vi "satellite simulator control.vi"() -> ()   [LabVIEW 2012]
uses:
  <vilib>/Utility/error.llb/DialogType.ctl
  <vilib>/DAQmx/create/channels.llb/DAQmx Create Channel (DO-Digital Output).vi
  <vilib>/Instr/_visa.llb/VISA Configure Serial Port (Instr).vi
  <vilib>/vision/NI_Vision_Development_Module.lvlib
  <vilib>/ptbypt/NI_PtbyPt.lvlib
panel:
  in  "Reaction Wheel":bool
  out "Write String":string
  in  "Control Value":sgl=1.5 format="%.4f"
  in  "Control Mode":u16(ring) items=["Idle"=0, "PWM (-1..1)"=1, "Current (-2.5..2.5A)"=2, "Speed (Rads/s)"=3, "Acceleration (Rads/sec^2)"=16, "Momentum (N-m-sec)"=17, "Torque (N-m)"=18]
  in  "Dst":i32=36 format="%x"
  in  "stop bits":u16(ring)=10 items=["1.0"=10, "1.5"=15, "2.0"=20]
  in  "VISA resource name (write)":refnum<visa-resource-name>="COM4"
  in  "flow control":u16(ring) items=["None"=0, "XON/XOFF"=1, "RTS/CTS"=2, "DTR/DSR"=4]
  in  "parity (0:none)":u16(ring) items=["None", "Odd", "Even", "Mark", "Space"]
  in  "data bits (8)":u16=8 min=5 max=8 step=1
  in  "baud rate (115200)":u32=115200
  out "bytes written":u32
  in  "bytes to read":u32=12
  out "Read string":string
  out "bytes read":u32
  out "Filtered Ohmega":dbl format="%0.2f"
  in  "VISA resource name":refnum<visa-resource-name>
  out "read buffer":string
  out "Ohmega":dbl[](graph)
  out "Filtered Ohmega":dbl[](graph)
  in  "Floating":bool
  in  "Thruster 8":bool
  in  "Thruster 7":bool
  in  "Thruster 6":bool
  in  "Thruster 5":bool
  in  "Thruster 4":bool
  in  "Thruster 3":bool
  in  "Thruster 2":bool
  in  "Truster1":bool
  in  "Thrusters Bundled":bool=TRUE
  in  "Manual Control Mode (Default)":bool
  in  "Up":bool
  in  "Right":bool
  in  "Down":bool
  in  "Left":bool
  in  "Stop 2":bool
  in  "CntrClk":bool
  in  "ClkWise":bool
  in  "Angular Acceleration":u16(ring) items=["Fast", "Slow"]
  in  "Duty Cycle":dbl=1.0
  in  "Automatic PD Position Controller":bool
  in  "Pixel-Distance Ratio (pix/cm)":dbl=8.26
  in  "Remote Logger Status":bool
  in  "Downlink Object Data?":bool
  in  "Remote Port":u16=61557
  in  "Local Port":u16=61556
  in  "Remote Host":string="localhost"
  in  "broadcast":bool
  in  "Maintain Attitude":bool
  out "alpha":dbl
  out "Objects":T1(array[cluster]) {"Aspect Ratio" format="%.2f"; "Orientation" format="%.2f"; "Area" format="%.2f"; "Object Center"."Y" format="%.2f"; "Object Center"."X" format="%.2f"}
  in  "Y Center Correction":dbl
  in  "X Center Correction":dbl
  out "Offset Degree":dbl
  in  "Y Desired":dbl
  in  "X Desired":dbl
  out "Vx (cm/s)":dbl
  out "Vy (cm/s)":dbl
  in  "OK Button":bool
  in  "Air Floating Status":bool
  in  "Control Freq":u32=20
  in  "Alpha Desired":dbl
  in  "STOP":bool caption="stop (F)"
  out "Image Out":T2(plugin-control)
  out "alpha (deg)":dbl
  out "dx (cm)":dbl
  out "dy (cm)":dbl
  # "Bundled Operations"
  # "Unbundled Operations"
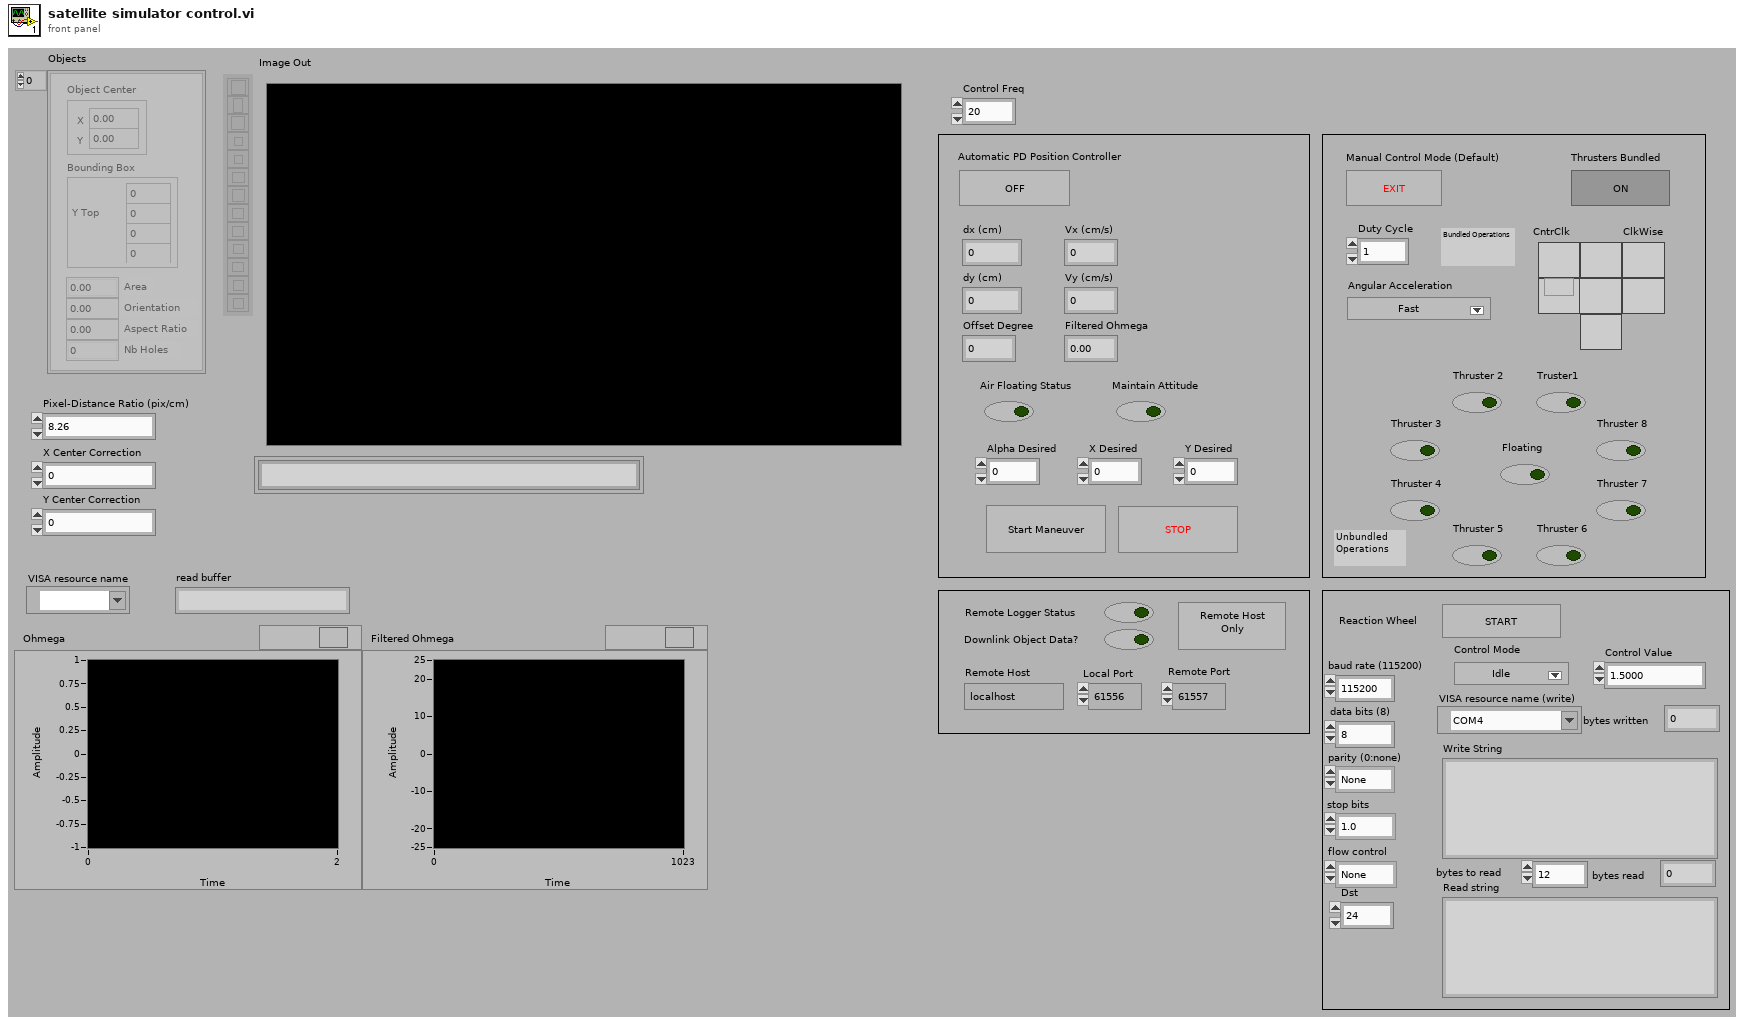
[diagram p1: front panel]
types:
  T1 = cluster{"Object Center":cluster{"X":sgl, "Y":sgl}, "Bounding Box":cluster{"X Left":i32, "Y Top":i32, "X Right":i32, "Y Bottom":i32}, "Area":sgl, "Orientation":sgl, "Aspect Ratio":sgl, "Nb Holes":i32}[]
  T2 = typedef "IMAQ Image.ctl" = refnum<image>
  T3 = typedef "DialogType.ctl" = u16
  T4 = cluster{"dx (cm)":dbl, "dy (cm)":dbl, "Offset Degree":dbl}
  T5 = cluster{"Objects":u16, "Threshold":i32, "Reject Border":bool, "Fill Holes":bool, "Min Object Size":bool, "Min Size":i32, "Max Object Size":bool, "Max Size":i32, "Show Search Area":bool, "Show Center":bool, "Show Bounding Box":bool}
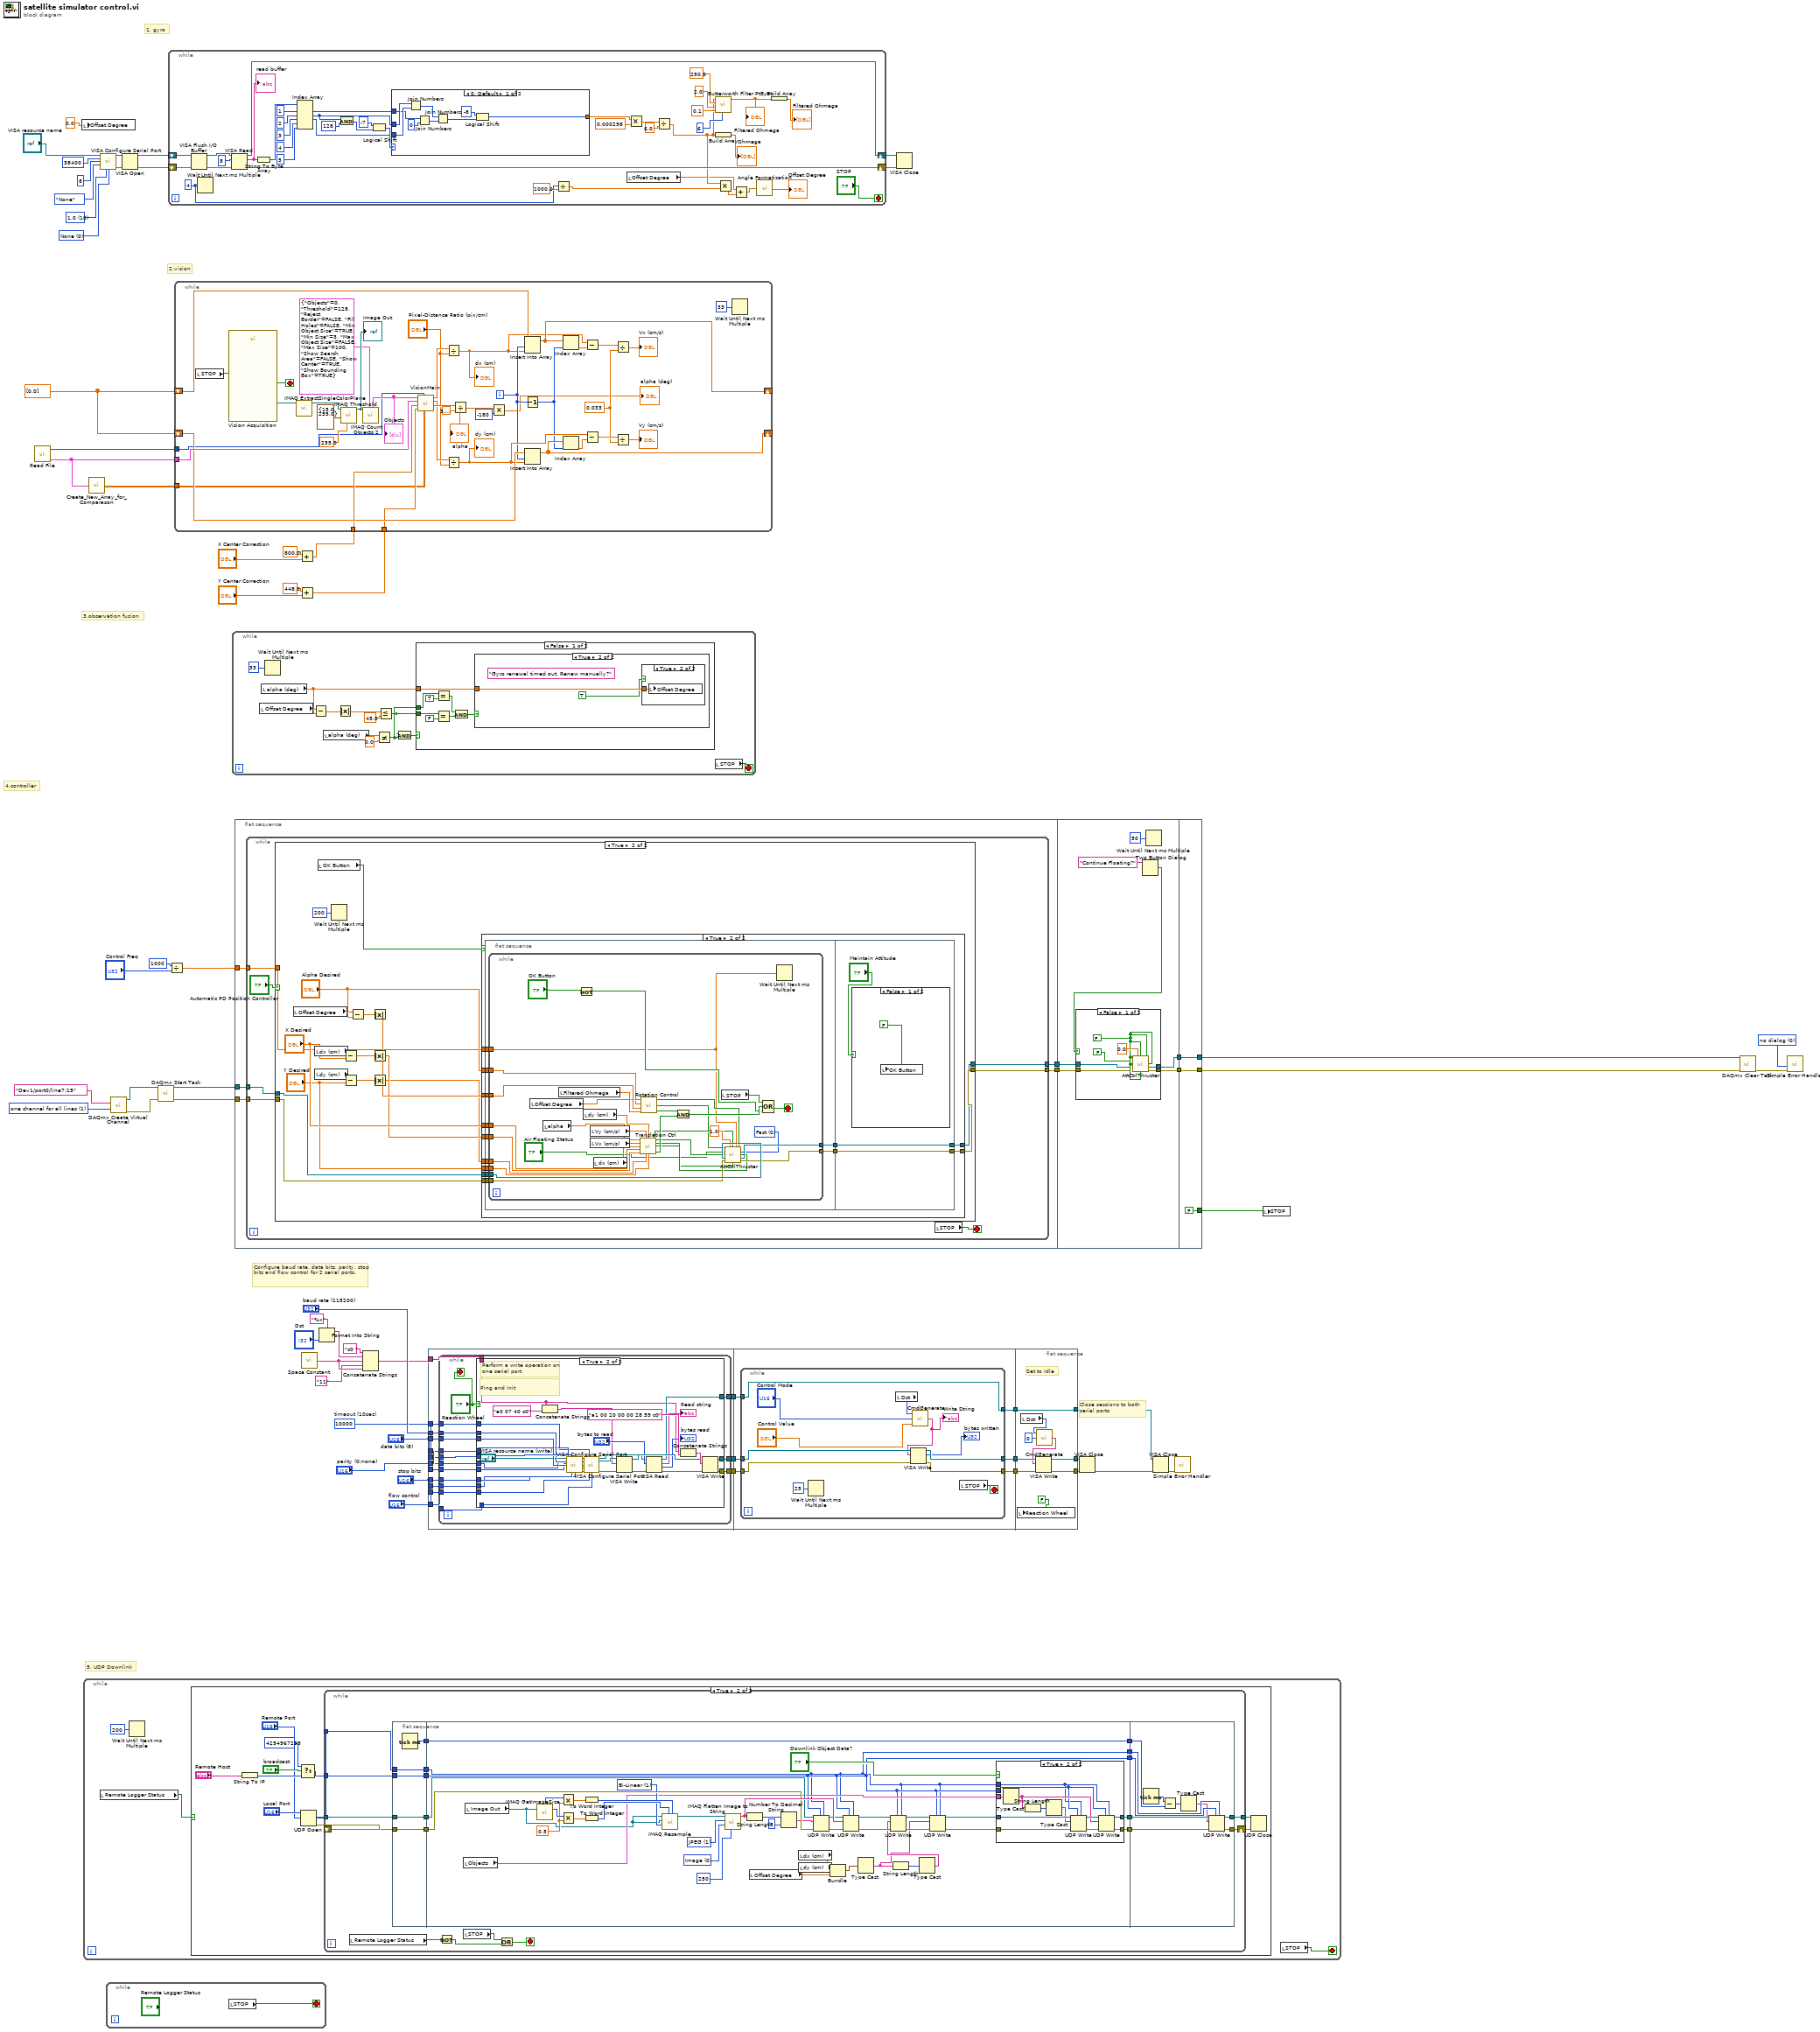
[diagram p0: block diagram]
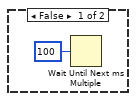
[diagram p2: hidden frame]
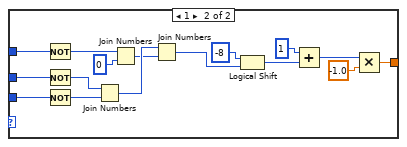
[diagram p3: hidden frame]
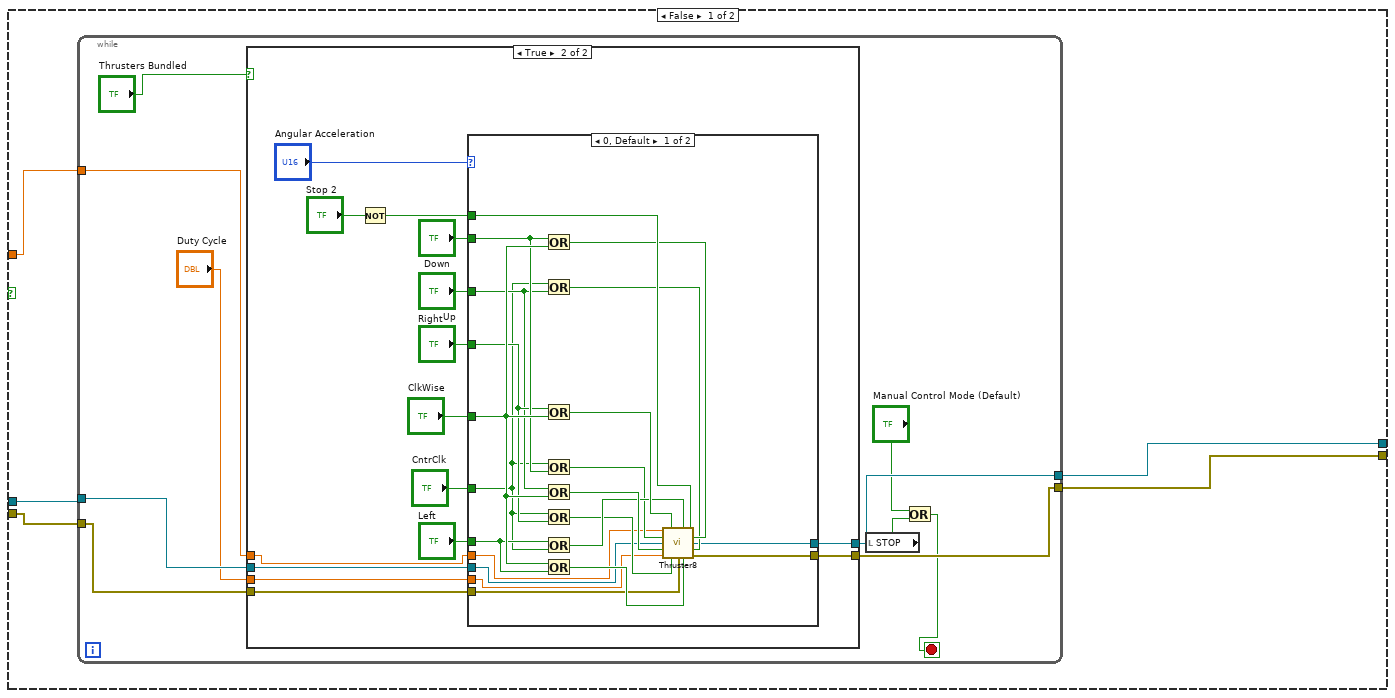
[diagram p6: hidden frame]
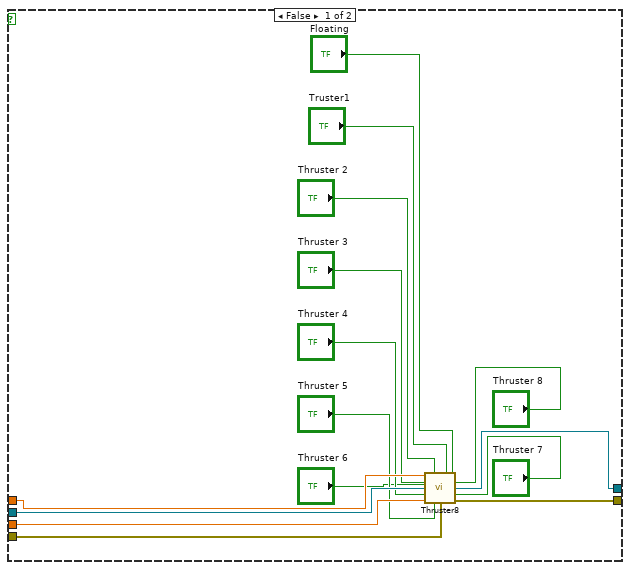
[diagram p7: hidden frame]
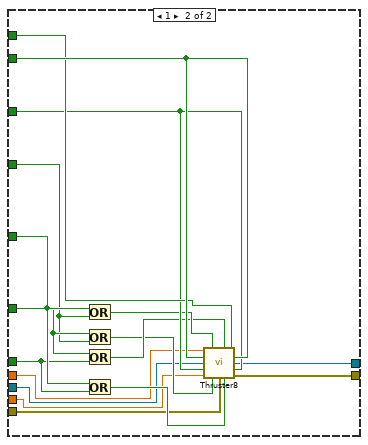
[diagram p8: hidden frame]
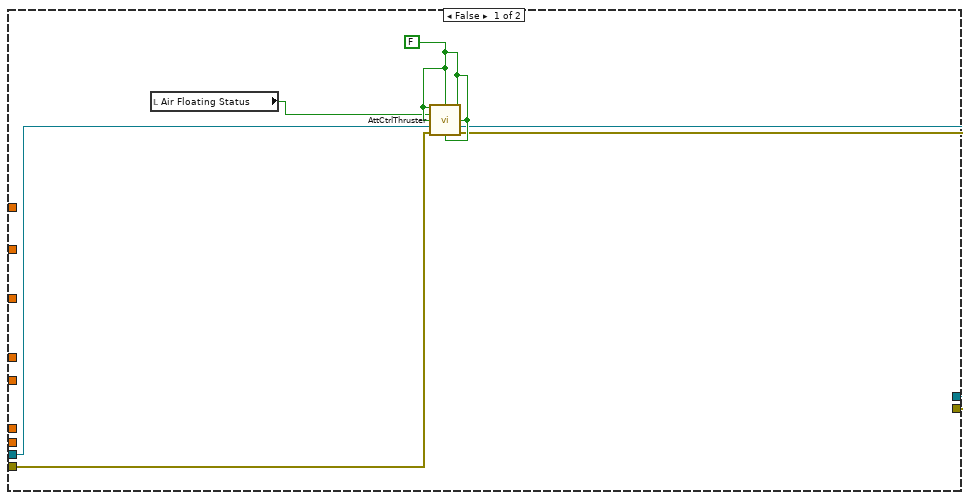
[diagram p9: hidden frame]
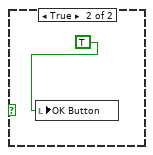
[diagram p10: hidden frame]
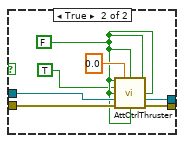
[diagram p11: hidden frame]
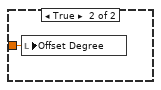
[diagram p14: hidden frame]
diagram:
  w15 = u32 10000  # timeout (10sec)
  w30 = u16 0 items=["None", "XON/XOFF", "RTS/CTS", "XON/XOFF & RTS/CTS", "DTR/DSR", "XON/XOFF & DTR/DSR"] ("flow control (0:none)")
  w32 = u16 10 items=["1.0"=10, "1.5"=15, "2.0"=20] ("stop bits (10: 1 bit)")
  w60 = T3 0 items=["no dialog", "OK message", "continue or stop message", "OK message + warnings", "continue/stop + warnings"] ("type of dialog (OK msg:1)")
  w63 = 1 items=["one channel for each line", "one channel for all lines"] ("line grouping")
  w49 = dbl[] [0.0]
  # "Close sessions to both serial ports"
  # "Configure baud rate, data bits, parity, stop bits and flow control for 2 serial ports."
  # "5. UDP Downlink"
  # "4.controller"
  # "3.observation fusion"
  # "2.vision"
  # "1. gyro"
  n1 = call "Read File.vi"() -> ("Objects"=w29:T1, "Total Obj"=w27:i32)  [unwired: 1 in]
  n2 = local write "Offset Degree"(0.0 ("y")) -> ()
  n3 = while {
    stop <- w67 stop-if-true
    n4 = local read "Remote Logger Status"() -> (w68:bool)
    n5 = Wait Until Next ms Multiple(millisecond multiple=u32 200) -> ()  [unwired: 1 out]
    n6 = case shown="True" w68 {
      frame False {
      }
      frame True {
        n7 = String To IP(1:"Remote Host") -> (0:w76:u32)
        n8 = Select(t=u32 4294967295, s="broadcast", f=w76) -> (s? t:f=w73:u32)
        n9 = UDP Open(11:"Local Port") -> (port=w72:refnum<k16>, 0:w71:errorcluster)  [unwired: 1 in, 4 out]
        n10 = while {
          tunnel: "Remote Port" -> [w99]
          tunnel: w73 -> [w98]
          tunnel: w72 -> [w97]
          tunnel: [w95] -> w70
          shift-right: [w94] -> w69
          shift-left: w71 -> [w96]
          stop <- w83 stop-if-true
          n11 = local read "Remote Logger Status"() -> (w81:bool)
          n12 = flat-sequence {
            tunnel: w97 -> [w101]
            tunnel: w99 -> [w102]
            tunnel: w98 -> [w103]
            tunnel: w96 -> [w104]
            tunnel: [w104] -> w93
            tunnel: [w103] -> w92
            tunnel: [w102] -> w91
            tunnel: [w101] -> w90
            tunnel: [w100] -> w89
            tunnel: [w124] -> w88
            tunnel: [w123] -> w87
            tunnel: w93 -> [w142]
            tunnel: w92 -> [w106]
            tunnel: w91 -> [w105]
            tunnel: w90 -> [w126]
            tunnel: [w125] -> w86
            tunnel: w89 -> [w125]
            tunnel: [w105] -> w85
            tunnel: [w106] -> w84
            tunnel: [w166] -> w95
            tunnel: [w160] -> w94
            tunnel: w88 -> [w161]
            tunnel: w87 -> [w167]
            tunnel: w86 -> [w168]
            tunnel: w85 -> [w165]
            tunnel: w84 -> [w164]
            frame #0 {
              n13 = Tick Count (ms)() -> (millisecond timer value=w100:u32)
            }
            frame #1 {
              w130 = u32 1 items=["Zero Order", "Bi-Linear", "Quadratic", "Cubic Spline"] ("Interpolation Type")
              w131 = 0.5
              w139 = 0 items=["Image", "Image and Vision Info", "Reference to Image"] ("Type of Flatten (Image and Vision Info)")
              w144 = 1 items=["None", "JPEG", "PACKED BINARY"] ("Compression (None)")
              n14 = local read "Objects"() -> (w121:T1)
              n15 = local read "Image Out"() -> (w120:T2)
              n16 = call "IMAQ GetImageSize"("Image"=w120) -> ("Y Resolution"=w132:i32, "X Resolution"=w133:i32)  [unwired: 3 in, 1 out]
              n17 = Multiply(x=w133, y=w131) -> (x*y=w135:dbl)
              n18 = Multiply(x=w132, y=w131) -> (x*y=w137:dbl)
              n19 = To Word Integer(number=w135) -> (16bit integer=w134:i16)
              n20 = To Word Integer(number=w137) -> (16bit integer=w136:i16)
              n21 = call "IMAQ Resample"("X Resolution"=w134, "Y Resolution"=w136, "Interpolation Type"=w130, "Image Dst"=w120, "Image Src"=w120) -> ("Image Dst Out"=w138:T2)  [unwired: 5 in, 1 out]
              n22 = call "IMAQ Flatten Image to String"("Quality (750)"=250, "Type of Flatten (Image and Vision Info)"=w139, "Compression (None)"=w144, "Image"=w138) -> ("Data String"=w143:string)  [unwired: 6 in, 1 out]
              n23 = String Length(string=w143) -> (length=w129:i32)
              n24 = local read "Offset Degree"() -> (w117:dbl)
              n25 = Number To Decimal String(number=w129, width (-)=i16 5) -> (decimal integer string=w128:string)
              n26 = local read "dx (cm)"() -> (w119:dbl)
              n27 = local read "dy (cm)"() -> (w118:dbl)
              n28 = UDP Write(address=w106, port or service name=w105, connection ID=w126, data in=w128, 8:w142) -> (error out=w141:errorcluster, 3:w140:refnum<k16>)  [unwired: 1 out]
              n29 = Bundle("dx (cm)"=w119, "dy (cm)"=w118, "Offset Degree"=w117) -> (w116:T4)  [unwired: 1 in]
              n30 = UDP Write(address=w106, port or service name=w105, connection ID=w140, data in=w143, 8:w141) -> (error out=w114:errorcluster, 3:w115:refnum<k16>)  [unwired: 1 out]
              n31 = Type Cast(x=w116) -> (*(type *) &x=w107:string)  [unwired: 1 in]
              n32 = String Length(string=w107) -> (length=w109:i32)
              n33 = Type Cast(x=w109) -> (*(type *) &x=w108:string)  [unwired: 1 in]
              n34 = UDP Write(address=w106, port or service name=w105, connection ID=w115, data in=w108, 8:w114) -> (error out=w113:errorcluster, 3:w111:refnum<k16>)  [unwired: 1 out]
              n35 = UDP Write(address=w106, port or service name=w105, connection ID=w111, data in=w107, 8:w113) -> (error out=w112:errorcluster, 3:w110:refnum<k16>)  [unwired: 1 out]
              n36 = case shown="True" "Downlink Object Data?" {
                tunnel: w121 -> [_ w159]
                tunnel: w112 -> [w147 w157]
                tunnel: [w147 w155] -> w124
                tunnel: w110 -> [w146 w154]
                tunnel: [w146 w152] -> w123
                tunnel: w106 -> [_ w149]
                tunnel: w105 -> [_ w148]
                frame False {
                }
                frame True {
                  n37 = Type Cast(x=w159) -> (*(type *) &x=w150:string)  [unwired: 1 in]
                  n38 = String Length(string=w150) -> (length=w158:i32)
                  n39 = Type Cast(x=w158) -> (*(type *) &x=w151:string)  [unwired: 1 in]
                  n40 = UDP Write(address=w149, port or service name=w148, connection ID=w154, data in=w151, 8:w157) -> (error out=w156:errorcluster, 3:w153:refnum<k16>)  [unwired: 1 out]
                  n41 = UDP Write(address=w149, port or service name=w148, connection ID=w153, data in=w150, 8:w156) -> (error out=w155:errorcluster, 3:w152:refnum<k16>)  [unwired: 1 out]
                }
              }
            }
            frame #2 {
              n42 = Tick Count (ms)() -> (millisecond timer value=w169:u32)
              n43 = Subtract(x=w169, y=w168) -> (x-y=w163:u32)
              n44 = Type Cast(x=w163) -> (*(type *) &x=w162:string)  [unwired: 1 in]
              n45 = UDP Write(address=w164, port or service name=w165, connection ID=w167, data in=w162, 8:w161) -> (error out=w160:errorcluster, 3:w166:refnum<k16>)  [unwired: 1 out]
            }
          }
          n46 = Not(x=w81) -> (.not. x?=w80:bool)
          n47 = local read "STOP"() -> (w82:bool)
          n48 = Or(x=w82, y=w80) -> (x .or. y?=w83:bool)
        }
        n49 = UDP Close(connection ID=w70, 8:w69) -> ()  [unwired: 2 out]
      }
    }
    n50 = local read "STOP"() -> (w67:bool)
  }
  n51 = call "Create_New_Array_for_Comparason.vi"("Captured Plots"=w29) -> ("Generated Distance Array"=w28:dbl[][])
  n52 = call-poly "VISA Configure Serial Port"("VISA resource name"="VISA resource name", "baud rate (9600)"=u32 38400, "data bits (8)"=u16 8, "parity (0:none)"=enum16{"None", "Odd", "Even", "Mark", "Space"}."None", "stop bits (10: 1 bit)"=w32, "flow control (0:none)"=w30) -> ("VISA resource name out"=w37:refnum<visa-resource-name>, "error out"=w36:errorcluster)  [unwired: 8 in]
  n53 = while {
    stop <- w170 stop-if-true
    n54 = local read "STOP"() -> (w170:bool)
  }
  n55 = call-poly <vilib>:"DAQmx Create Virtual Channel.vi"("lines"=tag "Dev1/port0/line7:15" ("Lines"), "line grouping"=w63) -> ("task out"=w61:refnum<k21>, "error out"=w62:errorcluster)  [unwired: 12 in]
  n56 = VISA Open(error in (no error)=w36, VISA resource name=w37) -> (VISA resource name=w35:refnum<visa-resource-name>, error out=w34:errorcluster)  [unwired: 3 in]
  n57 = call <vilib>:"DAQmx Start Task.vi"("task/channels in"=w61, "error in"=w62) -> ("task out"=w56:refnum<k21>, "error out"=w55:errorcluster)  [unwired: 12 in]
  n58 = while {
    shift-right: [w180] -> w3
    shift-left: w34 -> [w209]
    shift-right: [w181] -> w4
    shift-left: w35 -> [w210]
    stop <- "STOP" stop-if-true
    w172 = u32 4 ("millisecond multiple")
    n59 = VISA Flush I/O Buffer(VISA resource name=w210, error in (no error)=w209) -> (VISA resource name out=w208:refnum<visa-resource-name>, error out=w207:errorcluster)  [unwired: 1 in]
    n60 = Wait Until Next ms Multiple(millisecond multiple=w172) -> ()  [unwired: 1 out]
    n61 = VISA Read(VISA resource name=w208, byte count=u32 8, error in (no error)=w207) -> (VISA resource name out=w181:refnum<visa-resource-name>, read buffer=w182:string, error out=w180:errorcluster)  [unwired: 1 out]
    "read buffer" <- w182
    n62 = String To Byte Array(string=w182) -> (unsigned byte array=w203:u8[])
    n63 = Index Array(array=w203, index #1=1 ("index"), index #2=2 ("index"), index #3=3 ("index"), index #4=4 ("index"), index #5=5 ("index")) -> (element #1=w187:u8, element #2=w186:u8, element #3=w185:u8)  [unwired: 2 out]
    n64 = And(x=w186, y=u8 128) -> (x .and. y?=w197:u8)
    n65 = Logical Shift(y=i16 -7, x=w197) -> (x << y=w195:u8)
    n66 = case shown="0, Default" w195 {
      tunnel: [w212 w221] -> w199
      tunnel: w187 -> [w213 w231]
      tunnel: w186 -> [w215 w230]
      tunnel: w185 -> [w214 w229]
      frame 0, Default {
        n67 = Join Numbers(hi=w215, lo=w214) -> ((hi.lo)=w220:u16)
        n68 = Join Numbers(hi=w213, lo=u8 0) -> ((hi.lo)=w218:u16)
        n69 = Join Numbers(hi=w220, lo=w218) -> ((hi.lo)=w217:u32)
        n70 = Logical Shift(y=i16 -8, x=w217) -> (x << y=w212:u32)
      }
      frame 1 {
        n71 = Not(x=w231) -> (.not. x?=w226:u8)
        n72 = Not(x=w230) -> (.not. x?=w228:u8)
        n73 = Not(x=w229) -> (.not. x?=w227:u8)
        n74 = Join Numbers(hi=w228, lo=w227) -> ((hi.lo)=w236:u16)
        n75 = Join Numbers(hi=w226, lo=u8 0) -> ((hi.lo)=w234:u16)
        n76 = Join Numbers(hi=w236, lo=w234) -> ((hi.lo)=w233:u32)
        n77 = Logical Shift(y=i16 -8, x=w233) -> (x << y=w225:u32)
        n78 = Add(x=u32 1, y=w225) -> (x+y=w222:u32)
        n79 = Multiply(x=w222, y=-1.0) -> (x*y=w221:dbl)
      }
    }
    n80 = Divide(x=w172, y=1000.0) -> (x/y=w171:dbl)
    n81 = local read "Offset Degree"() -> (w177:dbl)
    n82 = Multiply(x=w199, y=0.000298) -> (x*y=w205:dbl)
    n83 = Divide(x=w205, y=6.0) -> (x/y=w178:dbl)
    n84 = call <vilib>:"Butterworth Filter PtByPt.vi"("order"=6, "low cutoff freq: fl"=0.1, "high cutoff freq: fh"=2.0, "sampling freq: fs"=250.0, "x"=w178) -> ("Filtered x"=w189:dbl)  [unwired: 4 in, 1 out]
    "Filtered Ohmega" <- w189
    n85 = Build Array(w178) -> (→"Ohmega":dbl[])
    n86 = Multiply(x=w178, y=w171) -> (x*y=w176:dbl)
    n87 = Add(x=w177, y=w176) -> (x+y=w175:dbl)
    n88 = call "Angle Formatization.vi"("Alpha"=w175) -> ("Alpha Formatized"=→"Offset Degree":dbl)
    n89 = Build Array(w189) -> (→"Filtered Ohmega":dbl[])
  }
  n90 = Divide(x=u32 1000 ("milliseconds to wait"), y="Control Freq") -> (x/y=w52:dbl)
  n91 = while {
    stop <- w247 stop-if-true
    n92 = local read "Offset Degree"() -> (w246:dbl)
    n93 = local read "alpha (deg)"() -> (w242:dbl)
    n94 = Wait Until Next ms Multiple(millisecond multiple=u32 33) -> ()  [unwired: 1 out]
    n95 = Subtract(x=w246, y=w242) -> (x-y=w245:dbl)
    n96 = local read "alpha (deg)"() -> (w240:dbl)
    n97 = Absolute Value(x=w245) -> (abs(x)=w244:dbl)
    n98 = Not Equal?(x=w240, y=0.0) -> (x != y?=w238:bool)
    n99 = Less Or Equal?(x=w244, y=45.0) -> (x <= y?=w237:bool)
    n100 = And(x=w237, y=w238) -> (x .and. y?=w241:bool)
    n101 = case shown="False" w241 {
      tunnel: w242 -> [w249 w260]
      tunnel: w238 -> [w251 _]
      tunnel: w237 -> [w250 _]
      frame False {
        n102 = Equal?(x=w251, y=TRUE) -> (x = y?=w255:bool)
        n103 = Equal?(x=w250, y=FALSE) -> (x = y?=w254:bool)
        n104 = And(x=w255, y=w254) -> (x .and. y?=w252:bool)
        n105 = case shown="True" w252 {
          tunnel: w249 -> [_ w258]
          frame False {
          }
          frame True {
            (unwired) "Gyro renewal timed out. Renew manually?" ("message")
            n106 = case shown="True" TRUE {
              tunnel: w258 -> [_ w259]
              frame False {
              }
              frame True {
                n107 = local write "Offset Degree"(w259) -> ()
              }
            }
          }
        }
      }
      frame True {
        n108 = local write "Offset Degree"(w260) -> ()
      }
    }
    n109 = local read "STOP"() -> (w247:bool)
  }
  n110 = flat-sequence {
    tunnel: w56 -> [w265]
    tunnel: w55 -> [w264]
    tunnel: w52 -> [w261]
    tunnel: [w263] -> w51
    tunnel: [w262] -> w50
    tunnel: w51 -> [w450]
    tunnel: w50 -> [w448]
    tunnel: [w449] -> w42
    tunnel: [w447] -> w41
    tunnel: [w466] -> w53
    tunnel: [w467] -> w54
    tunnel: w42 -> [w467]
    tunnel: w41 -> [w466]
    tunnel: [FALSE] -> w40
    frame #0 {
      n111 = while {
        tunnel: w265 -> [w272]
        tunnel: w264 -> [w271]
        tunnel: [w270] -> w263
        tunnel: [w269] -> w262
        tunnel: w261 -> [w267]
        stop <- w268 stop-if-true
        n112 = case shown="True" "Automatic PD Position Controller" {
          tunnel: w272 -> [w276 w374]
          tunnel: w271 -> [w275 w373]
          tunnel: [w273 w372] -> w270
          tunnel: [w274 w371] -> w269
          tunnel: w267 -> [w277 w357]
          frame False {
            n113 = while {
              tunnel: w277 -> [w287]
              tunnel: w276 -> [w286]
              tunnel: [w285] -> w274
              tunnel: [w284] -> w273
              tunnel: w275 -> [w283]
              stop <- w280 stop-if-true
              n114 = case shown="True" "Thrusters Bundled" {
                tunnel: w287 -> [w298 w310]
                tunnel: w286 -> [w302 w309]
                tunnel: [w299 w308] -> w285
                tunnel: [w300 w307] -> w284
                tunnel: w283 -> [w301 w306]
                tunnel: "Duty Cycle" -> [w297 w303]
                frame False {
                  n115 = call "Thruster8.vi"("period"=w298, "Thruster 2"="Thruster 2", "Truster1"="Truster1", "Floating"="Floating", "Thruster 3"="Thruster 3", "Thruster 8"="Thruster 8", "task in"=w302, "Thruster 4"="Thruster 4", "Thruster 7"="Thruster 7", "Duty Cycle"=w297, "Thruster 5"="Thruster 5", "error in"=w301, "Thruster 6"="Thruster 6") -> ("task out"=w299:refnum<k21>, "error out"=w300:errorcluster)  [unwired: 1 in]
                }
                frame True {
                  n116 = Not(x="Stop 2") -> (.not. x?=w304:bool)
                  n117 = case shown="0, Default" "Angular Acceleration" {
                    tunnel: w304 -> [w338 w354]
                    tunnel: "Down" -> [w330 w355]
                    tunnel: "Left" -> [w332 w348]
                    tunnel: "Up" -> [w326 w353]
                    tunnel: "Right" -> [w328 w346]
                    tunnel: "ClkWise" -> [w334 w352]
                    tunnel: "CntrClk" -> [w325 w349]
                    tunnel: w303 -> [w323 w344]
                    tunnel: w310 -> [w322 w343]
                    tunnel: w309 -> [w321 w339]
                    tunnel: [w320 w340] -> w308
                    tunnel: [w319 w341] -> w307
                    tunnel: w306 -> [w318 w342]
                    frame 0, Default {
                      n118 = Or(x=w330, y=w334) -> (x .or. y?=w333:bool)
                      n119 = Or(x=w325, y=w326) -> (x .or. y?=w324:bool)
                      n120 = Or(x=w328, y=w334) -> (x .or. y?=w336:bool)
                      n121 = Or(x=w325, y=w330) -> (x .or. y?=w329:bool)
                      n122 = Or(x=w326, y=w334) -> (x .or. y?=w337:bool)
                      n123 = Or(x=w325, y=w328) -> (x .or. y?=w327:bool)
                      n124 = Or(x=w332, y=w325) -> (x .or. y?=w331:bool)
                      n125 = Or(x=w334, y=w332) -> (x .or. y?=w335:bool)
                      n126 = call "Thruster8.vi"("period"=w322, "Thruster 2"=w336, "Truster1"=w331, "Floating"=w338, "Thruster 3"=w329, "Thruster 8"=w333, "task in"=w321, "Thruster 4"=w337, "Thruster 7"=w324, "Duty Cycle"=w323, "Thruster 5"=w327, "error in"=w318, "Thruster 6"=w335) -> ("task out"=w320:refnum<k21>, "error out"=w319:errorcluster)  [unwired: 1 in]
                    }
                    frame 1 {
                      n127 = Or(x=w352, y=w346) -> (x .or. y?=w351:bool)
                      n128 = Or(x=w349, y=w346) -> (x .or. y?=w345:bool)
                      n129 = Or(x=w349, y=w348) -> (x .or. y?=w347:bool)
                      n130 = Or(x=w352, y=w348) -> (x .or. y?=w350:bool)
                      n131 = call "Thruster8.vi"("period"=w343, "Thruster 2"=w351, "Truster1"=w347, "Floating"=w354, "Thruster 3"=w355, "Thruster 8"=w355, "task in"=w339, "Thruster 4"=w353, "Thruster 7"=w353, "Duty Cycle"=w344, "Thruster 5"=w345, "error in"=w342, "Thruster 6"=w350) -> ("task out"=w340:refnum<k21>, "error out"=w341:errorcluster)  [unwired: 1 in]
                    }
                  }
                }
              }
              n132 = local read "STOP"() -> (w282:bool)
              n133 = Or(x="Manual Control Mode (Default)", y=w282) -> (x .or. y?=w280:bool)
            }
          }
          frame True {
            n134 = local read "Offset Degree"() -> (w370:dbl)
            n135 = local read "dx (cm)"() -> (w366:dbl)
            n136 = local read "dy (cm)"() -> (w362:dbl)
            n137 = local read "OK Button"() -> (w358:bool)
            n138 = Wait Until Next ms Multiple(millisecond multiple=u32 200) -> ()  [unwired: 1 out]
            n139 = Subtract(x=w366, y="X Desired") -> (x-y=w364:dbl)
            n140 = Subtract(x=w362, y="Y Desired") -> (x-y=w360:dbl)
            n141 = Subtract(x=w370, y="Alpha Desired") -> (x-y=w368:dbl)
            n142 = Absolute Value(x=w368) -> (abs(x)=w367:dbl)
            n143 = Absolute Value(x=w364) -> (abs(x)=w363:dbl)
            n144 = Absolute Value(x=w360) -> (abs(x)=w359:dbl)
            n145 = case shown="True" w358 {
              tunnel: w374 -> [w378 w393]
              tunnel: w373 -> [w377 w392]
              tunnel: [w376 w391] -> w372
              tunnel: [w375 w390] -> w371
              tunnel: w357 -> [_ w389]
              tunnel: "Alpha Desired" -> [_ w388]
              tunnel: w367 -> [_ w387]
              tunnel: "X Desired" -> [_ w386]
              tunnel: w363 -> [_ w385]
              tunnel: "Y Desired" -> [_ w384]
              tunnel: w359 -> [_ w383]
              frame False {
                w380 = FALSE
                n146 = local read "Air Floating Status"() -> (w379:bool)
                n147 = call "AttCtrlThruster.vi"("ctclk"=w380, "Up"=w380, "clkwis"=w380, "Float"=w379, "Left"=w380, "Right"=w380, "task in"=w378, "error in"=w377, "Down"=w380) -> ("task out"=w375:refnum<k21>, "error out"=w376:errorcluster)  [unwired: 5 in]
              }
              frame True {
                n148 = flat-sequence {
                  tunnel: w393 -> [w404]
                  tunnel: w392 -> [w403]
                  tunnel: w389 -> [w400]
                  tunnel: w388 -> [w399]
                  tunnel: w387 -> [w398]
                  tunnel: w386 -> [w397]
                  tunnel: w385 -> [w396]
                  tunnel: w384 -> [w395]
                  tunnel: w383 -> [w394]
                  tunnel: [w402] -> w382
                  tunnel: [w401] -> w381
                  tunnel: [w440] -> w390
                  tunnel: [w441] -> w391
                  tunnel: w382 -> [w441]
                  tunnel: w381 -> [w440]
                  frame #0 {
                    n149 = while {
                      tunnel: w404 -> [w438]
                      tunnel: w403 -> [w437]
                      tunnel: [w435] -> w402
                      tunnel: [w436] -> w401
                      tunnel: w400 -> [w406]
                      tunnel: w399 -> [w416]
                      tunnel: w398 -> [w431]
                      tunnel: w397 -> [w415]
                      tunnel: w396 -> [w426]
                      tunnel: w395 -> [w414]
                      tunnel: w394 -> [w413]
                      stop <- w432 stop-if-true
                      w422 = u16 0 items=["Fast", "Slow"] ("Angular Acceleration")
                      n150 = local read "Offset Degree"() -> (w429:dbl)
                      n151 = local read "alpha"() -> (w410:dbl)
                      n152 = local read "Filtered Ohmega"() -> (w430:dbl)
                      n153 = Not(x="OK Button") -> (.not. x?=w411:bool)
                      n154 = local read "dy (cm)"() -> (w424:dbl)
                      n155 = local read "Vy (cm/s)"() -> (w425:dbl)
                      n156 = local read "Vx (cm/s)"() -> (w428:dbl)
                      n157 = local read "dx (cm)"() -> (w427:dbl)
                      n158 = call "Translation Ctrl.vi"("Alpha"=w410, "Filtered Speed Y"=w425, "Y In"=w424, "Filtered Speed X"=w428, "X In"=w427, "X Desired"=w415, "Original Difference X"=w426, "Original Difference Y"=w413, "Y Desired"=w414) -> ("Left"=w420:bool, "Right"=w419:bool, "Down"=w418:bool, "Up"=w417:bool, "Maneuver Complete?"=w421:bool)  [unwired: 2 in]
                      n159 = call "Rotation Control.vi"("Filtered Ohmega"=w430, "Original Difference"=w431, "Alpha Desired"=w416, "Alpha In"=w429) -> ("Maneuver Complete?"=w409:bool, "Counter-ClkWise Rot Ctrl"=w408:bool, "Clockwise Rot Ctrl"=w407:bool)
                      n160 = And(x=w409, y=w421) -> (x .and. y?=w423:bool)
                      n161 = local read "STOP"() -> (w433:bool)
                      n162 = call "AttCtrlThruster.vi"("ctclk"=w408, "Duty Cycle"=1.0, "Up"=w417, "Period"=w406, "clkwis"=w407, "Float"="Air Floating Status", "Angular Acceleration"=w422, "Left"=w420, "Right"=w419, "task in"=w438, "error in"=w437, "Down"=w418) -> ("task out"=w436:refnum<k21>, "error out"=w435:errorcluster)  [unwired: 2 in]
                      n163 = Compound Arithmetic op=OR(w433, w423, w411) -> (w432:bool)
                      n164 = Wait Until Next ms Multiple(millisecond multiple=w406) -> ()  [unwired: 1 out]
                    }
                  }
                  frame #1 {
                    n165 = case shown="False" "Maintain Attitude" {
                      frame False {
                        n166 = local write "OK Button"(FALSE) -> ()
                      }
                      frame True {
                        n167 = local write "OK Button"(TRUE) -> ()
                      }
                    }
                  }
                }
              }
            }
          }
        }
        n168 = local read "STOP"() -> (w268:bool)
      }
    }
    frame #1 {
      n169 = Two Button Dialog(message="Continue Floating?") -> (T button?=w444:bool)  [unwired: 2 in]
      n170 = case shown="False" w444 {
        tunnel: w450 -> [w453 w464]
        tunnel: [w451 w463] -> w449
        tunnel: w448 -> [w454 w462]
        tunnel: [w452 w461] -> w447
        frame False {
          w456 = FALSE
          n171 = call "AttCtrlThruster.vi"("ctclk"=w456, "Duty Cycle"=0.0, "Up"=w456, "clkwis"=w456, "Float"=FALSE, "Left"=w456, "Right"=w456, "task in"=w454, "error in"=w453, "Down"=w456) -> ("task out"=w452:refnum<k21>, "error out"=w451:errorcluster)  [unwired: 4 in]
        }
        frame True {
          w459 = FALSE
          n172 = call "AttCtrlThruster.vi"("ctclk"=w459, "Duty Cycle"=0.0, "Up"=w459, "clkwis"=w459, "Float"=TRUE, "Left"=w459, "Right"=w459, "task in"=w462, "error in"=w464, "Down"=w459) -> ("task out"=w461:refnum<k21>, "error out"=w463:errorcluster)  [unwired: 4 in]
        }
      }
      n173 = Wait Until Next ms Multiple(millisecond multiple=u32 50) -> ()  [unwired: 1 out]
    }
    frame #2 {
    }
  }
  n174 = Add(x=800.0 ("c_x"), y="X Center Correction") -> (x+y=w46:dbl)
  n175 = Add(x=448.0 ("c_y"), y="Y Center Correction") -> (x+y=w43:dbl)
  n176 = while {
    tunnel: w29 -> [w494]
    shift-right: [w491] -> _
    shift-left: w49 -> [w492]
    shift-right: [w480] -> _
    shift-left: w49 -> [w483]
    tunnel: w43 -> [w473]
    tunnel: w46 -> [w472]
    tunnel: w28 -> [w469]
    tunnel: w27 -> [w468]
    i -> [w482]
    stop <- w505 stop-if-true
    w476 = 0.033 ("y")
    n177 = local read "STOP"() -> (w496:bool)
    n178 = call "Vision Acquisition"("Stop (F)"=w496) -> ("Image Out"=w500:T2, "Stopped"=w505:bool)  [unwired: 24 in, 1 out]
    n179 = call "IMAQ ExtractSingleColorPlane"("Image Src"=w500) -> ("Image Dst Out"=w504:T2)  [unwired: 9 in, 1 out]
    n180 = call "IMAQ Threshold"("Replace Value"=sgl 255.0 ("replace value"), "Range"=cluster{"lower value":sgl, "upper value":sgl} {"lower value"=15.0, "upper value"=255.0} ("threshold"), "Image Src"=w504) -> ("Image Dst Out"=w501:T2)  [unwired: 7 in, 1 out]
    "Image Out" <- w501
    n181 = call "IMAQ Count Objects 2"("Settings"=T5 {"Objects"=0, "Threshold"=128, "Reject Border"=FALSE, "Fill Holes"=FALSE, "Min Object Size"=TRUE, "Min Size"=3, "Max Object Size"=FALSE, "Max Size"=100, "Show Search Area"=FALSE, "Show Center"=TRUE, "Show Bounding Box"=TRUE}, "Image"=w501) -> ("Objects"=w495:T1)  [unwired: 5 in, 4 out]
    "Objects" <- w495
    n182 = call "VisionMain.vi"("Generated Distance Array"=w469, "Database Total Points"=w468, "Y Center"=w473, "X Center"=w472, "Original Plots"=w494, "Plots Captured"=w495) -> ("alpha"=w493:dbl, "dy"=w489:dbl, "dx"=w484:dbl)  [unwired: 3 in]
    "alpha" <- w493
    n183 = Divide(x=w484, y="Pixel-Distance Ratio (pix/cm)") -> (x/y=w479:dbl)
    "dx (cm)" <- w479
    n184 = Divide(x=w489, y="Pixel-Distance Ratio (pix/cm)") -> (x/y=w488:dbl)
    "dy (cm)" <- w488
    n185 = Divide(x=w493, y=3.141592653589793) -> (x/y=w498:dbl)
    n186 = Multiply(x=w498, y=-180) -> (x*y=→"alpha (deg)":dbl)
    n187 = Insert Into Array(array=w483, index=w482, new element=w479) -> (w480:dbl[])
    n188 = Insert Into Array(array=w492, index=w482, new element=w488) -> (w491:dbl[])
    n189 = Decrement(x=w482) -> (x-1=w481:i32)
    n190 = Index Array(array=w480, index=w481) -> (element=w478:dbl)
    n191 = Index Array(array=w491, index=w481) -> (element=w490:dbl)
    n192 = Subtract(x=w479, y=w478) -> (x-y=w477:dbl)
    n193 = Subtract(x=w488, y=w490) -> (x-y=w487:dbl)
    n194 = Divide(x=w477, y=w476) -> (x/y=→"Vx (cm/s)":dbl)
    n195 = Divide(x=w487, y=w476) -> (x/y=→"Vy (cm/s)":dbl)
    n196 = Wait Until Next ms Multiple(millisecond multiple=u32 33) -> ()  [unwired: 1 out]
  }
  n197 = call <vilib>:"Space Constant.vi"() -> ("String"=w20:string)
  n198 = Format Into String(format string="%x", "Dst") -> (resulting string=w21:string)  [unwired: 2 in, 1 out]
  n199 = Concatenate Strings("c0 " ("string"), w21, w20, "11" ("string"), w20) -> (w10:string)
  n200 = flat-sequence {
    tunnel: [w507] -> w19
    tunnel: [w520] -> w18
    tunnel: [w519] -> w17
    tunnel: w15 -> [w518]
    tunnel: "stop bits" -> [w517]
    tunnel: "flow control" -> [w516]
    tunnel: "baud rate (115200)" -> [w515]
    tunnel: "data bits (8)" -> [w514]
    tunnel: "parity (0:none)" -> [w513]
    tunnel: w15 -> [w512]
    tunnel: "parity (0:none)" -> [w511]
    tunnel: "data bits (8)" -> [w510]
    tunnel: "stop bits" -> [w509]
    tunnel: "flow control" -> [w508]
    tunnel: w10 -> [w506]
    tunnel: w19 -> [w573]
    tunnel: w18 -> [w571]
    tunnel: w17 -> [w570]
    tunnel: [w572] -> w7
    tunnel: [w569] -> w6
    tunnel: [w568] -> w5
    tunnel: [w592] -> w8
    tunnel: [w591] -> w9
    tunnel: [w594] -> w24
    tunnel: w7 -> [w594]
    tunnel: w6 -> [w590]
    tunnel: w5 -> [w593]
    frame #0 {
      n201 = while {
        tunnel: [w536] -> w520
        tunnel: [w535] -> w519
        tunnel: w518 -> [w534]
        tunnel: w517 -> [w533]
        tunnel: w516 -> [w532]
        tunnel: w515 -> [w531]
        tunnel: w514 -> [w530]
        tunnel: w513 -> [w529]
        tunnel: w512 -> [w528]
        tunnel: w511 -> [w527]
        tunnel: w510 -> [w526]
        tunnel: w509 -> [w525]
        tunnel: w508 -> [w524]
        tunnel: [w523] -> w507
        tunnel: w506 -> [w522]
        stop <- "Reaction Wheel" stop-if-true
        n202 = case shown="True" "Reaction Wheel" {
          tunnel: [_ w555] -> w536
          tunnel: [_ w554] -> w535
          tunnel: w534 -> [_ w553]
          tunnel: w533 -> [_ w552]
          tunnel: w532 -> [_ w551]
          tunnel: w531 -> [_ w550]
          tunnel: w530 -> [_ w549]
          tunnel: w529 -> [_ w548]
          tunnel: w528 -> [_ w547]
          tunnel: w527 -> [_ w546]
          tunnel: w526 -> [_ w545]
          tunnel: w525 -> [_ w544]
          tunnel: w524 -> [_ w543]
          tunnel: [_ w542] -> w523
          tunnel: w522 -> [_ w539]
          frame False {
            n203 = Wait Until Next ms Multiple(millisecond multiple=u32 100) -> ()  [unwired: 1 out]
          }
          frame True {
            # "Perform a write operation on one serial port"
            # "Ping and Init"
            n204 = Concatenate Strings(w539, "a0 07 40 c0" ("string")) -> (w540:string)
            n205 = call-poly "VISA Configure Serial Port"("VISA resource name"="VISA resource name (write)", "timeout (10sec)"=w553, "baud rate (9600)"=w546, "data bits (8)"=w545, "stop bits (10: 1 bit)"=w552, "flow control (0:none)"=w551) -> ("VISA resource name out"=w556:refnum<visa-resource-name>, "error out"=w561:errorcluster)  [unwired: 3 in, 5 out]
            n206 = call-poly "VISA Configure Serial Port"("VISA resource name"="VISA resource name (write)", "timeout (10sec)"=w547, "baud rate (9600)"=w550, "data bits (8)"=w549, "parity (0:none)"=w548, "error in (no error)"=w561, "stop bits (10: 1 bit)"=w544, "flow control (0:none)"=w543) -> ("VISA resource name out"=w557:refnum<visa-resource-name>, "error out"=w562:errorcluster)  [unwired: 2 in, 4 out]
            n207 = VISA Write(VISA resource name=w556, write buffer=w540, error in (no error)=w562) -> (VISA resource name out=w564:refnum<visa-resource-name>, error out=w563:errorcluster)  [unwired: 1 out]
            n208 = VISA Read(VISA resource name=w557, byte count="bytes to read", error in (no error)=w563) -> (VISA resource name out=w542:refnum<visa-resource-name>, read buffer=→"Read string":string, return count=→"bytes read":u32, error out=w565:errorcluster)
            n209 = Concatenate Strings(w539, "a1 00 20 00 00 28 59 c0" ("string")) -> (w567:string)
            n210 = VISA Write(VISA resource name=w564, write buffer=w567, error in (no error)=w565) -> (VISA resource name out=w555:refnum<visa-resource-name>, error out=w554:errorcluster)  [unwired: 1 out]
          }
        }
      }
    }
    frame #1 {
      n211 = while {
        tunnel: w573 -> [w584]
        tunnel: [w584] -> w572
        tunnel: w571 -> [w583]
        tunnel: w570 -> [w582]
        tunnel: [w581] -> w569
        tunnel: [w580] -> w568
        stop <- w585 stop-if-true
        n212 = Wait Until Next ms Multiple(millisecond multiple=u32 25) -> ()  [unwired: 1 out]
        n213 = local read "Dst"() -> (w579:i32)
        n214 = call "CmdGenerate.vi"("Control Value"="Control Value", "Mode"="Control Mode", "Dst"=w579) -> ("CMD code"=w575:string)
        "Write String" <- w575
        n215 = VISA Write(VISA resource name=w583, write buffer=w575, error in (no error)=w582) -> (VISA resource name out=w580:refnum<visa-resource-name>, return count=→"bytes written":u32, error out=w581:errorcluster)
        n216 = local read "STOP"() -> (w585:bool)
      }
    }
    frame #2 {
      # "Set to Idle"
      n217 = local write "Reaction Wheel"(FALSE) -> ()
      n218 = local read "Dst"() -> (w589:i32)
      n219 = call "CmdGenerate.vi"("Mode"=0, "Dst"=w589) -> ("CMD code"=w587:string)  [unwired: 1 in]
      n220 = VISA Write(VISA resource name=w593, write buffer=w587, error in (no error)=w590) -> (VISA resource name out=w592:refnum<visa-resource-name>, error out=w591:errorcluster)  [unwired: 1 out]
    }
  }
  n221 = VISA Close(VISA resource name=w4, error in (no error)=w3) -> ()  [unwired: 1 out]
  n222 = VISA Close(VISA resource name=w8, error in (no error)=w9) -> (error out=w26:errorcluster)
  n223 = VISA Close(VISA resource name=w24, error in (no error)=w26) -> (error out=w25:errorcluster)
  n224 = call <vilib>:"Simple Error Handler.vi"("error in (no error)"=w25) -> ()  [unwired: 1 in, 8 out]
  n225 = local write "STOP"(w40) -> ()
  n226 = call <vilib>:"DAQmx Clear Task.vi"("task in"=w53, "error in"=w54) -> ("error out"=w59:errorcluster)  [unwired: 13 in]
  n227 = call <vilib>:"Simple Error Handler.vi"("type of dialog (OK msg:1)"=w60, "error in (no error)"=w59) -> ()  [unwired: 3 in, 5 out]
